vi "comicvine.to.local_volume.vi"(5 "volume":i32, 7 "volume type":T1=enum."One Shot" caption="Enum", 8 "error in (no error)":errorcluster, 11 "cv volume":T2) -> (0 "error out":errorcluster, 3 "local volume":T6={"id"=0, "name"="", "sortable_name"="", "aliases"=[], "description"="", "site_detail_url"="", "count_of_issues"=0, "start_year"=0, "publisher_id"=0, "issue_ids"=[], "date_last_updated"=timestamp(0 s since 1904-01-01), "volume"=0, "cv_id"="", "volume type"=enum."One Shot"})   [LabVIEW 2024]
uses:
  definitions/local_volume.ctl
  definitions/volume.type--enum.ctl
  definitions/comicvine_volume.ctl
  definitions/comicvine_volume.results.ctl
  definitions/comicvine_volume.issue.ctl
  definitions/comicvine_volume.publisher.ctl
  <vilib>/Utility/error.llb/Trim Whitespace One-Sided.vi
  <userlib>/_OpenG.lib/string/string.llb/openg_string.lvlib
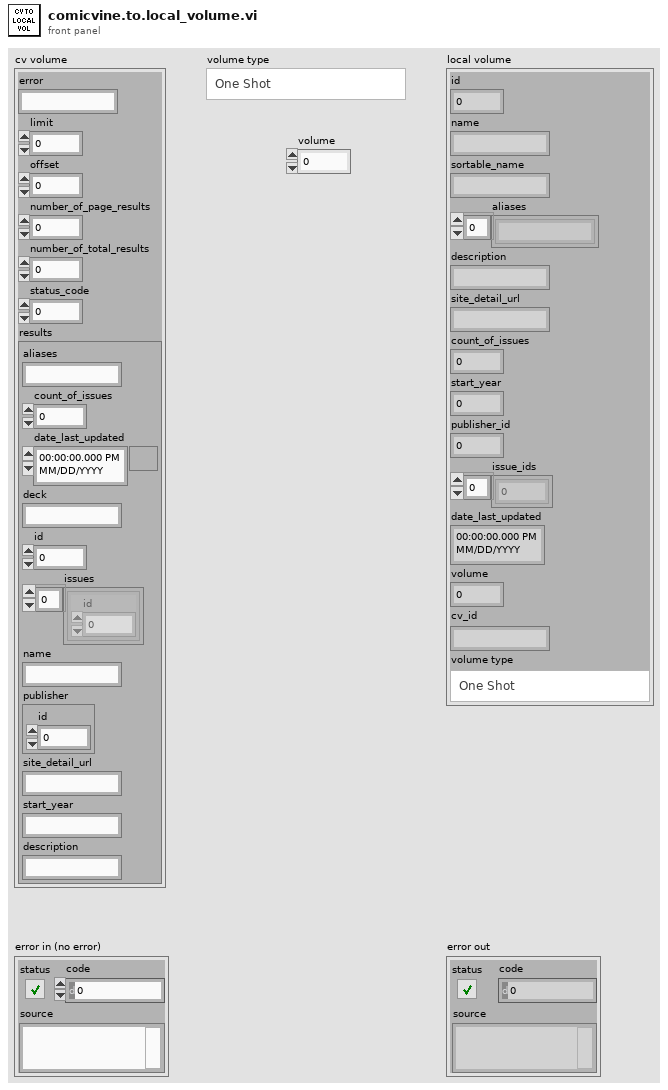
[diagram p1: front panel]
types:
  T1 = typedef "volume.type--enum.ctl" = enum16{"Ongoing", "Limited Series", "Annual", "One Shot", "Reprint/Document", "Star Comics", "Epic Comics"}
  T2 = typedef "comicvine_volume.ctl" = cluster{"error":string, "limit":i32, "offset":i32, "number_of_page_results":i32, "number_of_total_results":i32, "status_code":i32, "results":T3}
  T3 = typedef "comicvine_volume.results.ctl" = cluster{"aliases":string, "count_of_issues":i32, "date_last_updated":timestamp, "deck":string, "id":i32, "issues":T4[], "name":string, "publisher":T5, "site_detail_url":string, "start_year":string, "description":string}
  T4 = typedef "comicvine_volume.issue.ctl" = cluster{"id":i32}
  T5 = typedef "comicvine_volume.publisher.ctl" = cluster{"id":i32}
  T6 = typedef "local_volume.ctl" = cluster{"id":i32, "name":string, "sortable_name":string, "aliases":string[], "description":string, "site_detail_url":string, "count_of_issues":i32, "start_year":i32, "publisher_id":i32, "issue_ids":i32[], "date_last_updated":timestamp, "volume":i32, "cv_id":string, "volume type":T1}
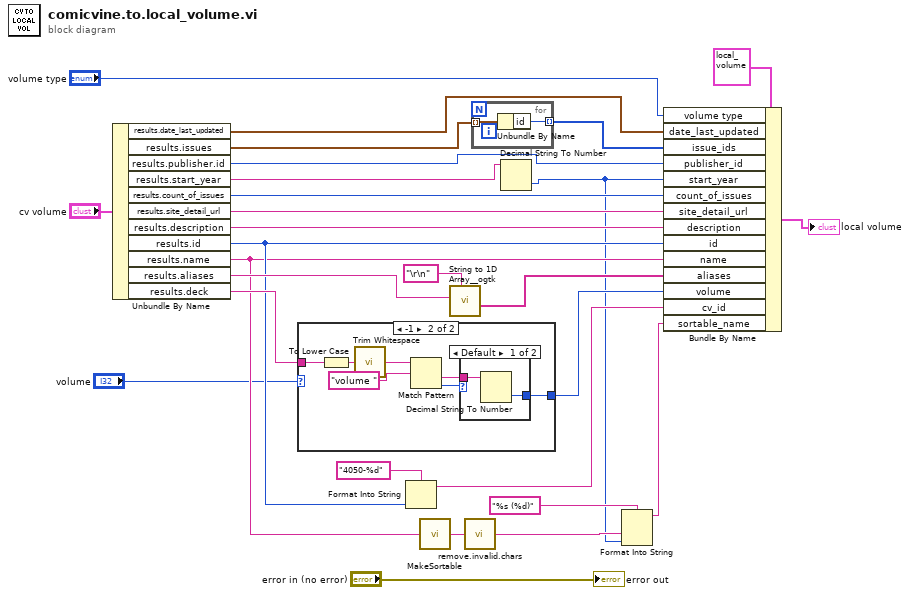
[diagram p0: block diagram]
diagram:
  n1 = Unbundle By Name("cv volume") -> ("results.date_last_updated"=w14:timestamp, "results.issues"=w16:T4[], "results.publisher.id"=w17:i32, "results.start_year"=w18:string, "results.count_of_issues"=w19:i32, "results.site_detail_url"=w20:string, "results.description"=w21:string, "results.id"=w10:i32, "results.name"=w7:string, "results.aliases"=w24:string, "results.deck"=w13:string)
  n2 = case shown="-1" "volume" {
    selector: "volume" -> [w29 _]
    tunnel: w13 -> [_ w36]
    tunnel: [w29 w30] -> w12
    frame Default {
    }
    frame -1 {
      n3 = To Lower Case(string=w36) -> (all lower case string=w35:string)
      n4 = call <vilib>:"Trim Whitespace.vi"("string"=w35) -> ("trimmed string"=w34:string)  [unwired: 1 in]
      n5 = Match Pattern(string=w34, regular expression="volume ") -> (after substring=w31:string, offset past match=w32:i32)  [unwired: 1 in, 2 out]
      n6 = case shown="Default" w32 {
        tunnel: w31 -> [w38 _]
        tunnel: [w37 _] -> w30
        frame Default {
          n7 = Decimal String To Number(string=w38) -> (number=w37:i32)  [unwired: 2 in, 1 out]
        }
        frame -1 {
        }
      }
    }
  }
  n8 = Format Into String(format string="4050-%d", w10) -> (resulting string=w9:string)  [unwired: 2 in, 1 out]
  n9 = call "MakeSortable.vi"("string in"=w7) -> ("string out"=w25:string)
  n10 = call <userlib>:"String to 1D Array__ogtk.vi"("delimiter (Tab)"="\r\n", "string"=w24) -> ("Array of Strings"=w22:string[])  [unwired: 9 in]
  n11 = call "remove.invalid.chars.vi"("string in"=w25) -> ("string out"=w4:string)
  n12 = for {
    tunnel: w16 -> [w40] mode=indexing
    tunnel: [w39] -> w15 mode=indexing
    n13 = Unbundle By Name(w40) -> ("id"=w39:i32)
  }
  n14 = Decimal String To Number(string=w18) -> (number=w3:i32)  [unwired: 2 in, 1 out]
  n15 = Format Into String(format string="%s (%d)", w4, w3) -> (resulting string=w2:string)  [unwired: 2 in, 1 out]
  n16 = Bundle By Name(cluster=T6 {"id"=0, "name"="", "sortable_name"="", "aliases"=[], "description"="", "site_detail_url"="", "count_of_issues"=0, "start_year"=0, "publisher_id"=0, "issue_ids"=[], "date_last_updated"=timestamp(0 s since 1904-01-01), "volume"=0, "cv_id"="", "volume type"=enum."One Shot"} ("volume"), "volume type"="volume type", "date_last_updated"=w14, "issue_ids"=w15, "publisher_id"=w17, "start_year"=w3, "count_of_issues"=w19, "site_detail_url"=w20, "description"=w21, "id"=w10, "name"=w7, "aliases"=w22, "volume"=w12, "cv_id"=w9, "sortable_name"=w2) -> (→"local volume":T6)
  "error out" <- "error in (no error)"
